vi "ReftoDVR--SMO.vi"(10 "Ref":u64 format="%016x") -> (2 "Ref":T1)   [LabVIEW 2021, in "smo.lvlib" / "SMO.lvclass"]
uses:
  SMO.lvclass
  Typedefs/PrivateData--Ref.ctl
  Typedefs/PrivateData--Cluster.ctl
  Typedefs/Parent Call--Enum.ctl
  Typedefs/RegisteredProcessData--Cluster.ctl
  Typedefs/Process Error Notification--Cluster.ctl
  Typedefs/Protected Events.ctl
  Typedefs/StopProcessEventData--Cluster.ctl
  Typedefs/AbortProcessEventData--Cluster.ctl
  Typedefs/SMO Dependency Event--Cluster.ctl
  Typedefs/SMO Dependency Event--Enum.ctl
  Typedefs/Public Events.ctl
  Typedefs/SMOState --Enum.ctl
  Typedefs/Reserve State--Enum.ctl
  Typedefs/Accessibility--Cluster.ctl
  SMO.lvclass/SMO.ctl
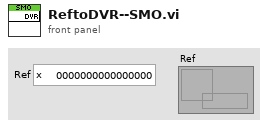
[diagram p1: front panel]
types:
  T1 = typedef "smo.lvlib/SMO.lvclass/PrivateData--Ref.ctl" = refnum<data-value>
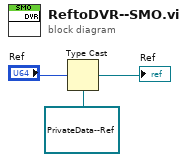
[diagram p0: block diagram]
diagram:
  n1 = Type Cast(type=T1 refnum ("data value reference"), x="Ref") -> (*(type *) &x=→"Ref":T1)
